vi "Ballard XML Generator.Open Message Buffers.vi"(11 "string in":string) -> (3 "string out":string)   [LabVIEW 2020]
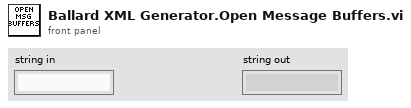
[diagram p1: front panel]
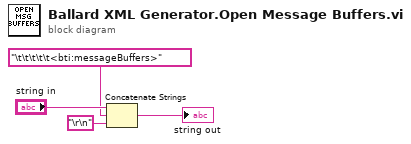
[diagram p0: block diagram]
diagram:
  n1 = Concatenate Strings("string in", "\t\t\t\t\t<bti:messageBuffers>", "\r\n") -> (→"string out":string)
